vi "Disconnect.vi"(1 "error in (no error)":errorcluster caption="Fehler (Eingang, kein Fehler)", 2 "lLSID":i32) -> (0 "error out":errorcluster caption="Fehler (Ausgang)")   [LabVIEW 2018, in "TangoOWN.lvlib"]
uses:
  TangoOWN.lvlib
  SDK/Tango.lvlib
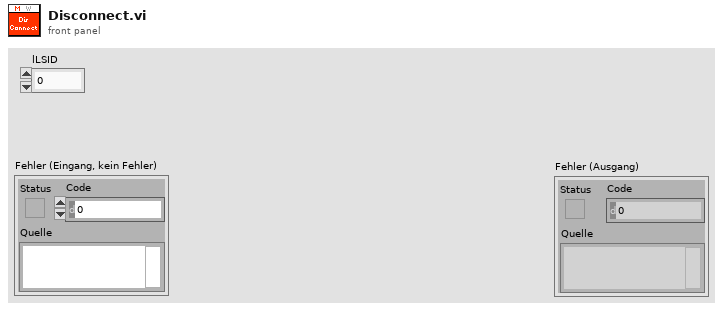
[diagram p1: front panel]
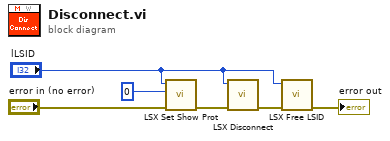
[diagram p0: block diagram]
diagram:
  n1 = call "LSX Set Show Prot.vi"("error in (no error)"="error in (no error)", "bShowProt"=0, "lLSID"="lLSID") -> ("error out"=w4:errorcluster)  [unwired: 7 in, 1 out]
  n2 = call "LSX Disconnect.vi"("error in (no error)"=w4, "lLSID"="lLSID") -> ("error out"=w6:errorcluster)  [unwired: 8 in, 1 out]
  n3 = call "LSX Free LSID.vi"("error in (no error)"=w6, "lLSID"="lLSID") -> ("error out"=→"error out":errorcluster)  [unwired: 8 in, 1 out]
